vi "Select Players Dialog.vi"(8 "error in (no error)":errorcluster, 11 "Reversi in":refnum<class "Reversi.lvclass">) -> (0 "error out":errorcluster, 3 "Reversi out":refnum<class "Reversi.lvclass">)   [LabVIEW 2020, in "Reversi.lvlib" / "Reversi.lvclass"]
uses:
  Reversi.lvclass
  aa9f3d6a-4b9f-455d-bcc5-b1d428e522bf.vi
  edd00b8c-893c-4bab-b4e2-fb96aafeb1a1.vi
panel:
  in  "White":string(combo)
  in  "Black":string(combo)
  in  "Start":bool
  # "Choose Players"
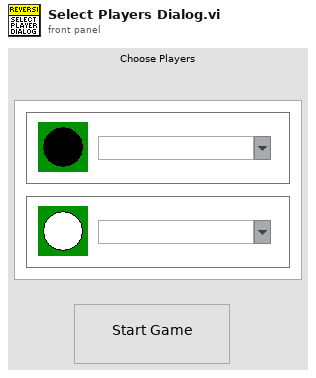
[diagram p1: front panel]
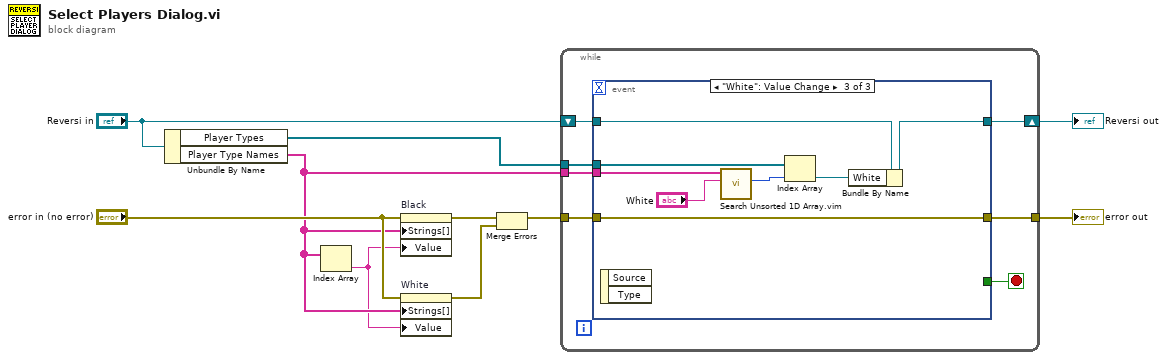
[diagram p0: block diagram]
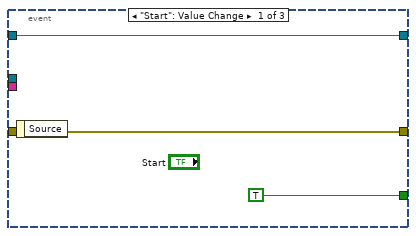
[diagram p2: hidden frame]
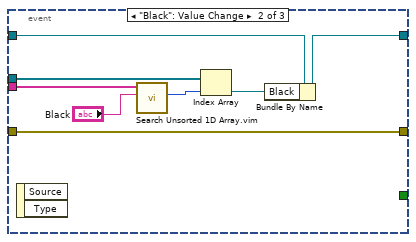
[diagram p3: hidden frame]
diagram:
  n1 = Unbundle By Name("Reversi in") -> ("Player Types"=w4:refnum<class "Player.lvclass">[], "Player Type Names"=w2:string[])
  n2 = Index Array(array=w2) -> (element=w1:string)  [unwired: 1 in]
  n3 = property on="Black" class="CmbBox"(error in="error in (no error)", "Strings[]"=w2, "Value"=w1) -> (error out=w9:errorcluster)  [unwired: 1 in, 1 out]
  n4 = property on="White" class="CmbBox"(error in="error in (no error)", "Strings[]"=w2, "Value"=w1) -> (error out=w6:errorcluster)  [unwired: 1 in, 1 out]
  n5 = Merge Errors(w9, w6) -> (w7:errorcluster)
  n6 = while {
    shift-right: [w15] -> w10
    shift-left: "Reversi in" -> [w17]
    tunnel: w4 -> [w13]
    tunnel: w2 -> [w14]
    tunnel: w7 -> [w12]
    tunnel: [w11] -> w5
    stop <- w16 stop-if-true
    n7 = event shown="[2] \"White\": Value Change" {
      selector: _ -> [_ _ _]
      dyn-events: _ -> [_ _ _]
      timeout: _ -> [_ _ _]
      tunnel: w17 -> [w20 w23 w32]
      tunnel: [TRUE _ _] -> w16
      tunnel: [w20 w24 w33] -> w15
      tunnel: w14 -> [_ w28 w36]
      tunnel: w13 -> [_ w26 w35]
      tunnel: w12 -> [w18 w21 w29]
      tunnel: [w18 w21 w29] -> w11
      event "Start": Value Change {
        n8 = event-data() -> ()  [unwired: 1 in, 1 out]
      }
      event "Black": Value Change {
        n9 = event-data() -> ()  [unwired: 1 in, 2 out]
        n10 = call "Search Unsorted 1D Array.vim"("element"="Black", "unsorted 1D array"=w28) -> ("index of element"=w25:i32)  [unwired: 9 in]
        n11 = Index Array(array=w26, index=w25) -> (element=w22:refnum<class "Player.lvclass">)
        n12 = Bundle By Name(cluster=w23, "Black"=w22) -> (w24:refnum<class "Reversi.lvclass">)
      }
      event "White": Value Change {
        n13 = event-data() -> ()  [unwired: 1 in, 2 out]
        n14 = call "Search Unsorted 1D Array.vim"("element"="White", "unsorted 1D array"=w36) -> ("index of element"=w34:i32)  [unwired: 9 in]
        n15 = Index Array(array=w35, index=w34) -> (element=w31:refnum<class "Player.lvclass">)
        n16 = Bundle By Name(cluster=w32, "White"=w31) -> (w33:refnum<class "Reversi.lvclass">)
      }
    }
  }
  "error out" <- w5
  "Reversi out" <- w10
